vi "Part Indices.vi"(10 "i":i32, 11 "Last Index":i32) -> (1 "Next Index":i32, 2 "Prev Index":i32, 3 "Index":i32)   [LabVIEW 2020, in "Stream.lvlib" / "URLPattern.lvclass"]
uses:
  URLPattern.lvclass
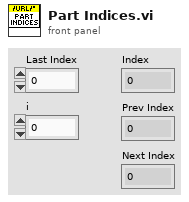
[diagram p1: front panel]
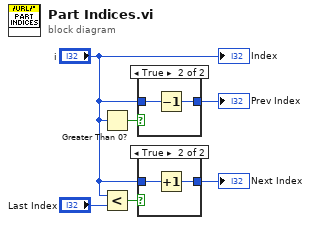
[diagram p0: block diagram]
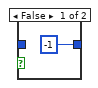
[diagram p2: hidden frame]
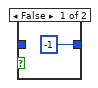
[diagram p3: hidden frame]
diagram:
  n1 = Greater Than 0?(x="i") -> (x > 0?=w3:bool)
  n2 = Less?(x="i", y="Last Index") -> (x < y?=w5:bool)
  n3 = case shown="True" w3 {
    tunnel: "i" -> [_ w9]
    tunnel: [-1 w8] -> w1
    frame False {
    }
    frame True {
      n4 = Decrement(x=w9) -> (x-1=w8:i32)
    }
  }
  "Prev Index" <- w1
  n5 = case shown="True" w5 {
    tunnel: "i" -> [_ w12]
    tunnel: [-1 w11] -> w4
    frame False {
    }
    frame True {
      n6 = Increment(x=w12) -> (x+1=w11:i32)
    }
  }
  "Next Index" <- w4
  "Index" <- "i"
